vi "Store Start Time.vi"(11 "Timestamp":dbl) -> ()   [LabVIEW 2014, in "CAN Bus Monitor Engine.lvlib"]
uses:
  BM Global Vars.vi
  CAN Bus Monitor Engine.lvlib
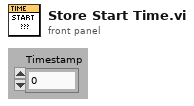
[diagram p1: front panel]
types:
  T1 = cluster{"IncMinFrameTime":dbl, "IncMaxFrameTime":dbl, "Min Frame Length":dbl[][], "Max Frame Length":dbl[][], "Std Frames":u32, "Ext Frames":u32, "Error Frames":u32, "Remote Frames":u32, "Std Frames / Sec":u32, "Ext Frames / Sec":u32, "Error Frames / Sec":u32, "Remote Frames / Sec":u32, "Peak Bus Load":dbl, "Bus Load":dbl, "Start Timestamp":dbl, "Null Frames":u32, "Null Frames / Sec":u32}
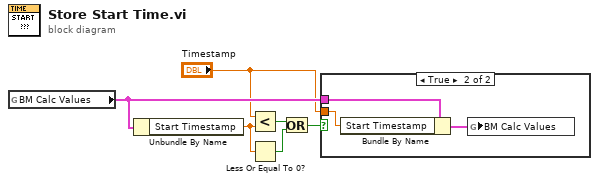
[diagram p0: block diagram]
diagram:
  n1 = global read "BM Global Vars.vi" "BM Calc Values"() -> (w6:T1)
  n2 = Unbundle By Name(w6) -> ("Start Timestamp"=w3:dbl)
  n3 = Less?(x="Timestamp", y=w3) -> (x < y?=w2:bool)
  n4 = Less Or Equal To 0?(x=w3) -> (x <= 0?=w5:bool)
  n5 = Or(x=w2, y=w5) -> (x .or. y?=w4:bool)
  n6 = case shown="True" w4 {
    tunnel: w6 -> [_ w9]
    tunnel: "Timestamp" -> [_ w7]
    frame False {
    }
    frame True {
      n7 = Bundle By Name(cluster=w9, "Start Timestamp"=w7) -> (w8:T1)
      n8 = global write "BM Global Vars.vi" "BM Calc Values"(w8) -> ()
    }
  }
